vi "Get All SubVi nodes in diagram.vi"(8 "error in":errorcluster, 11 "Diagram In":refnum<vi>) -> (0 "error out":errorcluster, 2 "All Sub-vis":refnum<vi>[](array[refnum]), 3 "Diagram Out":refnum<vi>, 4 "Vi Names":string[](array[string]), 5 "Vi-Refs":refnum<vi>[](array[refnum]))   [LabVIEW 2012, in "Scripting Tools.lvlib"]
doc: "Returns all Sub-Vi nodes from the block diagram referenced by <B>Diagram In</B>, including all those in sub-diagrams (loops and sequence structures etc). Also returns references to and names of all the sub-vis corresponding to the sub-vi nodes. If a sub-vi is called in more than one node, only one reference and name is returned."
uses:
  Scripting Tools.lvlib
  <vilib>/Utility/traverseref.llb/TRef TravTarget.ctl
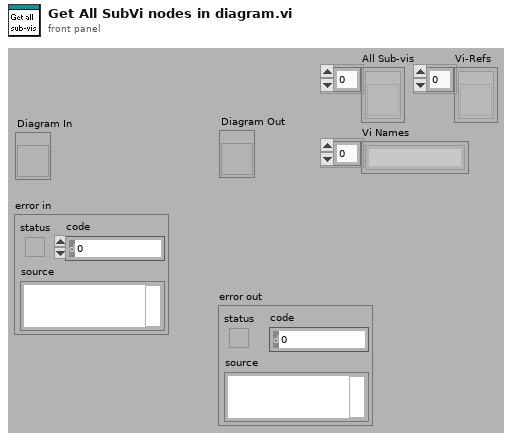
[diagram p1: front panel]
types:
  T1 = typedef "TRef TravTarget.ctl" = enum16{"FP", "BD", "Other"}
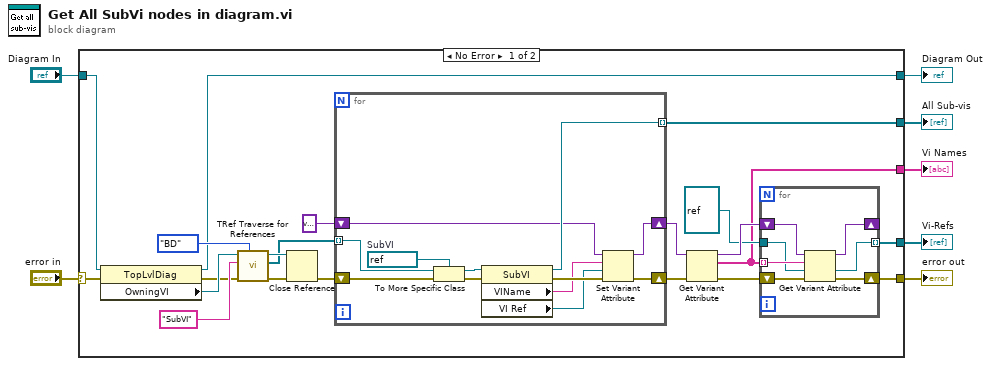
[diagram p0: block diagram]
diagram:
  n1 = case shown="No Error" "error in" {
    selector: "error in" -> [w28 w49]
    tunnel: "Diagram In" -> [w27 w48]
    tunnel: [w8 w49] -> w6
    tunnel: [w22 w48] -> w5
    tunnel: [w16 _] -> w3
    tunnel: [w10 _] -> w2
    tunnel: [w9 _] -> w1
    frame No Error {
      n2 = property class="TopLvlDiag"(reference=w27, error in=w28) -> (reference out=w22:refnum<vi>, error out=w23:errorcluster, "OwningVI"=w26:refnum<vi>)
      n3 = call <vilib>:"TRef Traverse for References.vi"("Traverse Target"=TRef_TravTarget."BD", "error in (no error)"=w23, "Class Name"="SubVI", "VI Refnum"=w26) -> ("error out"=w21:errorcluster, "References"=w18:refnum<vi>[], "dup VI Refnum"=w20:refnum<vi>)  [unwired: 1 in, 4 out]
      n4 = Close Reference(reference=w20, error in (no error)=w21) -> (error out=w19:errorcluster)
      n5 = for {
        shift-right: [w39] -> w14
        shift-left: w19 -> [w46]
        tunnel: w18 -> [w43] mode=indexing
        tunnel: [w42] -> w16 mode=indexing
        shift-right: [w37] -> w15
        shift-left: variant -> [w36]
        w47 = refnum<vi> refnum  # SubVI
        n6 = To More Specific Class(target class=w47, reference=w43, error in=w46) -> (specific class reference=w44:refnum<vi>, error out=w45:errorcluster)
        n7 = property class="SubVI"(reference=w44, error in=w45) -> (reference out=w42:refnum<vi>, error out=w41:errorcluster, "VIName"=w40:string, "VI Ref"=w38:refnum<vi>)
        n8 = Set Variant Attribute(Variant=w36, name=w40, value=w38, error in=w41) -> (Variant out=w37:variant, error out=w39:errorcluster)  [unwired: 1 out]
      }
      n9 = Get Variant Attribute(Variant=w15, error in=w14) -> (duplicate Variant=w12:variant, names=w10:string[], error out=w13:errorcluster)  [unwired: 3 out]
      n10 = for {
        tunnel: w10 -> [w33] mode=indexing
        shift-right: [w31] -> _
        shift-left: w12 -> [w34]
        shift-right: [w32] -> w8
        shift-left: w13 -> [w35]
        tunnel: refnum<vi> refnum ("vi reference") -> [w30]
        tunnel: [w29] -> w9 mode=indexing
        n11 = Get Variant Attribute(Variant=w34, name=w33, default value (empty Variant)=w30, error in=w35) -> (duplicate Variant=w31:variant, value=w29:refnum<vi>, error out=w32:errorcluster)  [unwired: 1 out]
      }
    }
    frame Error {
    }
  }
  "error out" <- w6
  "Diagram Out" <- w5
  "All Sub-vis" <- w3
  "Vi-Refs" <- w1
  "Vi Names" <- w2
